vi "发送数据处理.vi"(8 "error in (no error)":errorcluster caption="错误输入（无错误）", 10 "表格":string[][](table), 11 "基站":string(combo)) -> (0 "error out":errorcluster caption="错误输出", 2 "Submit TX":string, 3 "Bind TX":string)   [LabVIEW 2016, in "数据传输系统-02.lvlib"]
panel:
  in  "Bind 消息头":string="\u0016\u0000\u0000\u0000\u0001\u0000\u0000\u0000"
  out "Bind 基站标识号":string="05911015" caption="Bind 消息头"
  in  "Bind 密码":string="123456"
  in  "Submit 消息去向":string="05919999"
  out "Submit 消息内容的长度":string
  out "Submit 消息头":string
  out "Submit 消息来源":string="05911014"
  out "Submit 消息内容":string
  in  "Submit 保留2":string="\u0000\u0000\u0000\u0000"
  in  "Submit 应答标志位":string="\u0001"
  in  "Submit 保留1":string="\u0000\u0000\u0000\u0000"
  in  "F1":string=":"
  out "F2":string="05911014"
  in  "F3":string="@001"
  out "F4":string="20170716163000"
  out "F5":string="Z055.1234"
  in  "F6":string="FF"
  in  "F7":string="&"
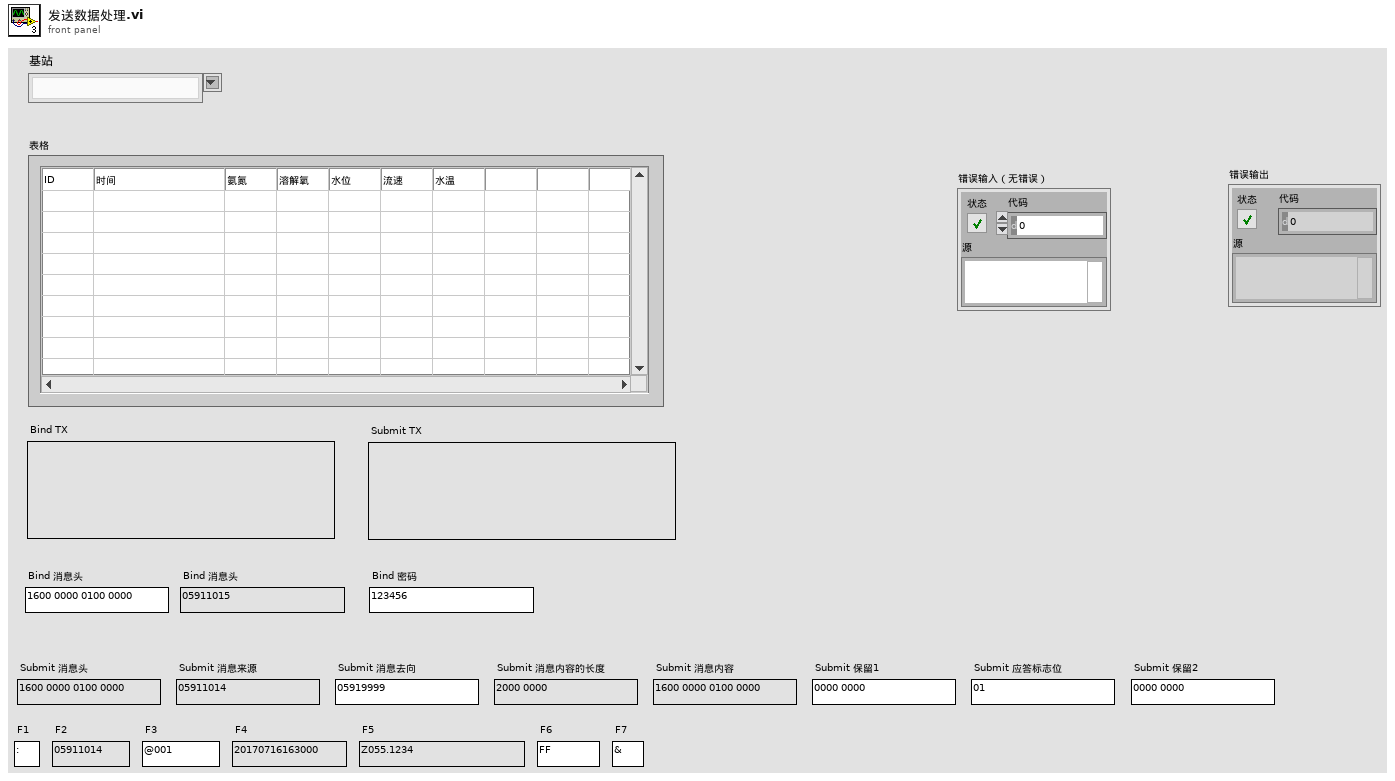
[diagram p1: front panel]
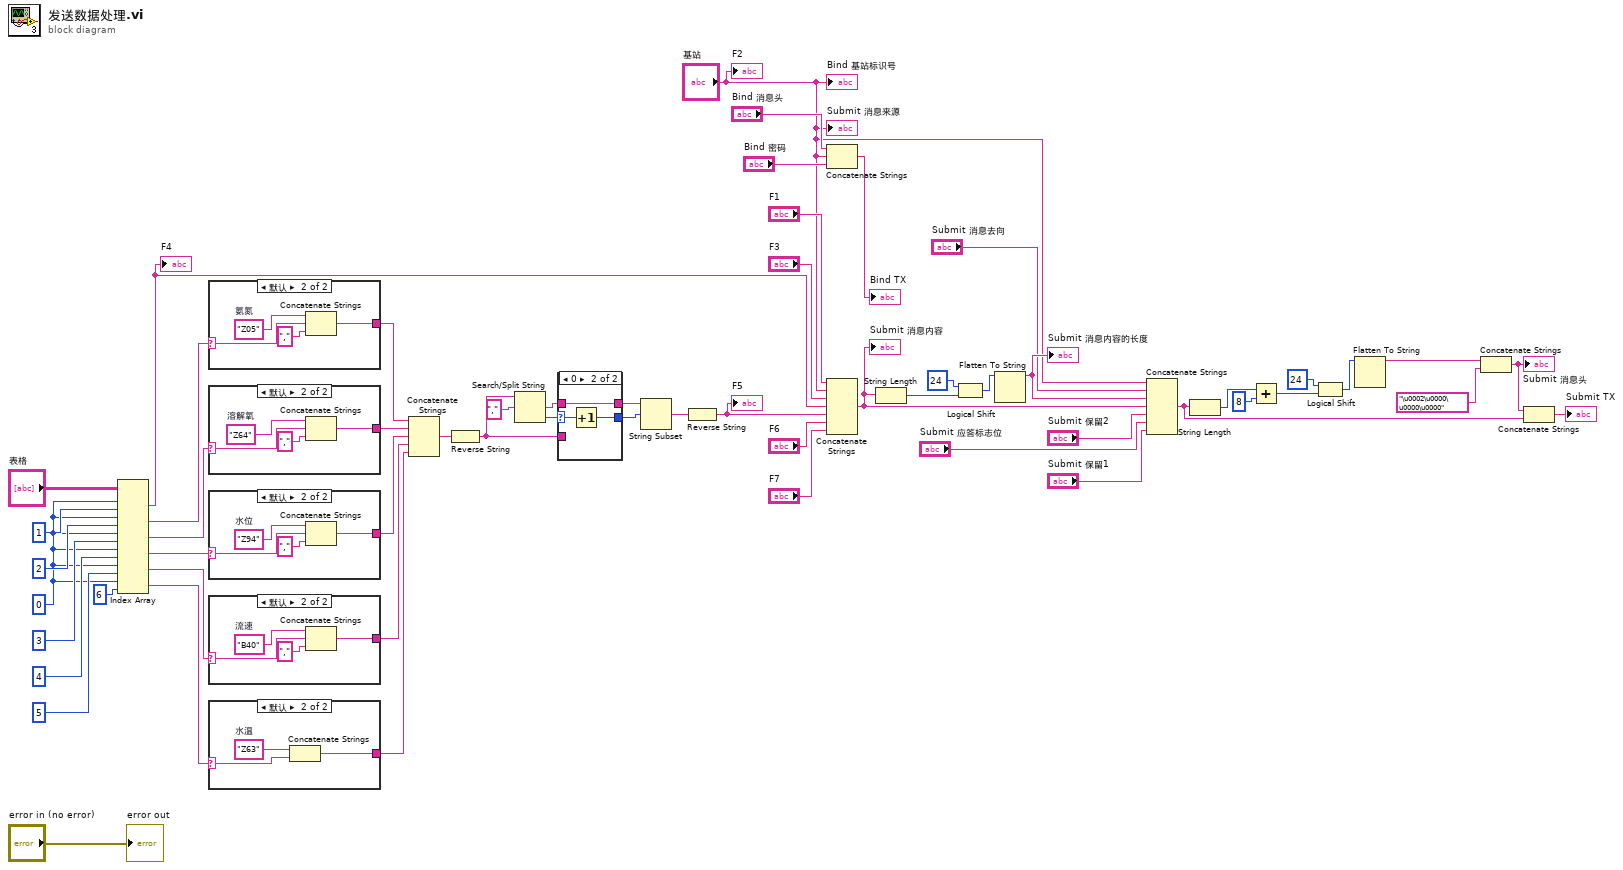
[diagram p0: block diagram]
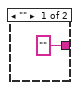
[diagram p3: hidden frame]
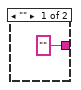
[diagram p4: hidden frame]
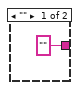
[diagram p5: hidden frame]
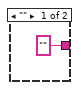
[diagram p6: hidden frame]
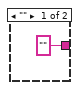
[diagram p7: hidden frame]
diagram:
  w19 = 0 ("索引 (行)")
  n1 = Index Array(array="表格", index (row) #1=w19, index (col) #1=1 ("禁用的索引 (列)"), index (row) #2=w19, index (col) #2=2 ("禁用的索引 (列)"), index (row) #3=w19, index (col) #3=3 ("禁用的索引 (列)"), index (row) #4=w19, index (col) #4=4 ("禁用的索引 (列)"), index (row) #5=w19, index (col) #5=5 ("禁用的索引 (列)"), index (row) #6=w19, index (col) #6=6 ("禁用的索引 (列)")) -> (element #1=w30:string, element #2=w15:string, element #3=w14:string, element #4=w13:string, element #5=w12:string, element #6=w11:string)
  "F4" <- w30
  n2 = case shown="默认" w15 {
    selector: w15 -> [_ w59]
    tunnel: ["" w60] -> w35
    frame "" {
    }
    frame Default {
      w61 = "Z05"  # 氨氮
      n3 = Concatenate Strings(w61, w59, "," ("字符串")) -> (w60:string)
    }
  }
  n4 = case shown="默认" w14 {
    selector: w14 -> [_ w63]
    tunnel: ["" w65] -> w36
    frame "" {
    }
    frame Default {
      w66 = "Z64"  # 溶解氧
      n5 = Concatenate Strings(w66, w63, "," ("字符串")) -> (w65:string)
    }
  }
  n6 = case shown="默认" w13 {
    selector: w13 -> [_ w69]
    tunnel: ["" w70] -> w17
    frame "" {
    }
    frame Default {
      w71 = "Z94"  # 水位
      n7 = Concatenate Strings(w71, w69, "," ("字符串")) -> (w70:string)
    }
  }
  n8 = case shown="默认" w12 {
    selector: w12 -> [_ w74]
    tunnel: ["" w75] -> w16
    frame "" {
    }
    frame Default {
      w76 = "B40"  # 流速
      n9 = Concatenate Strings(w76, w74, "," ("字符串")) -> (w75:string)
    }
  }
  n10 = case shown="默认" w11 {
    selector: w11 -> [_ w78]
    tunnel: ["" w79] -> w1
    frame "" {
    }
    frame Default {
      w80 = "Z63"  # 水温
      n11 = Concatenate Strings(w80, w78) -> (w79:string)
    }
  }
  n12 = Concatenate Strings(w35, w36, w17, w16, w1) -> (w10:string)
  n13 = Reverse String(1:w10) -> (0:w3:string)
  n14 = Search/Split String(string=w3, search string/char (-)="," ("字符串")) -> (match + rest of string=w4:string, offset of match=w5:i32)  [unwired: 1 in, 1 out]
  n15 = case shown="0" w5 {
    selector: w5 -> [_ w83]
    tunnel: [_ w84] -> w8
    tunnel: w4 -> [_ w82]
    tunnel: w3 -> [w81 _]
    tunnel: [w81 w82] -> w2
    frame Default {
    }
    frame 0 {
      n16 = Increment(x=w83) -> (x+1=w84:i32)
    }
  }
  n17 = String Subset(string=w2, offset (0)=w8) -> (substring=w7:string)  [unwired: 1 in]
  n18 = Reverse String(1:w7) -> (0:w6:string)
  "F5" <- w6
  n19 = Concatenate Strings("Bind 消息头", "基站", "Bind 密码") -> (→"Bind TX":string)
  n20 = Concatenate Strings("F1", "基站", "F3", w30, w6, "F6", "F7") -> (w39:string)
  "Submit 消息内容" <- w39
  n21 = String Length(string=w39) -> (length=w47:i32)
  n22 = Logical Shift(y=i16 24, x=w47) -> (x << y=w45:i32)
  n23 = Flatten To String(anything=w45) -> (data string=w40:string)  [unwired: 3 in, 2 out]
  "Submit 消息内容的长度" <- w40
  n24 = Concatenate Strings("基站", "Submit 消息去向", w40, w39, "Submit 保留2", "Submit 应答标志位", "Submit 保留1") -> (w25:string)
  n25 = String Length(string=w25) -> (length=w29:i32)
  n26 = Add(x=w29, y=8) -> (x+y=w27:i32)
  n27 = Logical Shift(y=i16 24, x=w27) -> (x << y=w44:i32)
  n28 = Flatten To String(anything=w44) -> (data string=w41:string)  [unwired: 3 in, 2 out]
  n29 = Concatenate Strings(w41, "\u0002\u0000\u0000\u0000" ("F7")) -> (w26:string)
  "Submit 消息头" <- w26
  n30 = Concatenate Strings(w26, w25) -> (→"Submit TX":string)
  "Bind 基站标识号" <- "基站"
  "Submit 消息来源" <- "基站"
  "F2" <- "基站"
  "error out" <- "error in (no error)"
